vi "LowEnd-FPGA.vi"() -> ()   [LabVIEW 2016]
uses:
  Faraday Cup Readback.ctl
  Aperture Readback.ctl
  Gate Valve Readback.ctl
  Glassman Control.ctl
  Glassman Readback.ctl
  <vilib>/LabVIEW Targets/FPGA/cRIO/shared/nicrio_ModuleControls/nicrio_cRIO-9871_BaudRateEnum.ctl
  <vilib>/LabVIEW Targets/FPGA/cRIO/shared/nicrio_ModuleControls/nicrio_cRIO-9871_DataBitsEnum.ctl
  <vilib>/LabVIEW Targets/FPGA/cRIO/shared/nicrio_ModuleControls/nicrio_cRIO-9871_ParityEnum.ctl
  <vilib>/LabVIEW Targets/FPGA/cRIO/shared/nicrio_ModuleControls/nicrio_cRIO-9871_StopBitsEnum.ctl
  <vilib>/Platform/TimedLoop/XDataNode/timing_clust.ctl
  <vilib>/Platform/TimedLoop/XDataNode/nitl_modes.ctl
  <vilib>/Platform/TimedLoop/XDataNode/wakeup.ctl
  <vilib>/rvi/FXPMathLib/basic elements/FxpIntAccumulator/subVIs/nifxpmath_IntAccumulator_SimConfig.ctl
  <vilib>/rvi/Emulation/niFpgaGetClockAttributes.vi
  <vilib>/rvi/Emulation/niFpgaSctlEmulationGetInTimedLoop.vi
  <vilib>/rvi/Emulation/niFpgaEmulationReportErrorSimple.vi
  <vilib>/rvi/eio/common/nirviEmuTemplateMethod_errors.vi
  <vilib>/rvi/Emulation/niFpgaCriticalErrorInLSC.vi
  <vilib>/rvi/Analysis/common/codeGenErrors/XNode/niFpgaXNodeCodeGenErrorHandle.vi
  <vilib>/rvi/FXPMathLib/basic elements/FxpIntAccumulator/simVIs/DllFxpIntAccumulator_sub.vi
  <vilib>/rvi/eio/common/nirviEmuTemplatePropertySet_errors.vi
  <vilib>/eio/EIONode/EIONode.xnode
  <vilib>/rvi/Analysis/measure/dc-rms/XNode/niFpgaDC-RMS.xnode
  <vilib>/Platform/TimedLoop/XDataNode/XDataNode.xnode
  <vilib>/rvi/FXPMathLib/basic elements/FxpIntAccumulator/XNode/nifxpmath_IntAccumulator.xnode
  <vilib>/rvi/FXPMathLib/FxpMul/XNode/nifxpmath_Multiplier.xnode
  <vilib>/eio/EIOPropertyNode/EIOPropertyNode.xnode
  <vilib>/eio/EIOMethodNode/EIOMethodNode.xnode
  <vilib>/Platform/TimedLoop/XDataNode/XDNodeRunTimeDep.lvlib
  <vilib>/rvi/FXPMathLib/sim/FxpSim.dll
  <vilib>/rvi/eio/common/nirviEmuTemplatePropertyGet_errors.vi
  <vilib>/rvi/eio/common/nirviEmuTemplatePropertyGet_noerrors.vi
  <vilib>/rvi/eio/common/nirviEmuTemplatePropertySet_noerrors.vi
panel:
  in  "Tank Entrance Vac Interlock bypass":bool
  in  "LowEnd Waist Vac Interlock bypass":bool
  out "HV readback loop #2 error":errorcluster
  out "Tank Entrance Y2- readback":T1
  out "Tank Entrance Y2+ readback":T1
  out "Tank Entrance Y1- readback":T1
  out "Tank Entrance Y1+ readback":T1
  out "Tank Entrance X- readback":T1
  out "Tank Entrance X+ readback":T1
  out "HV readback loop #1 error":errorcluster
  out "LE Einzel readback":T1
  out "LE Waist Y- readback":T1
  out "LE Waist Y+ readback":T1
  out "LE Waist X- readback":T1
  out "LE Waist X+ readback":T1
  out "HV control loop 1 error":errorcluster
  in  "LE Einzel V set":T2
  in  "LE Waist Y- Steerer V set":T2
  in  "LE Waist Y+ Steerer V set":T2
  in  "LE Waist X- Steerer V set":T2
  in  "LE Waist X+ Steerer V set":T2
  out "HV control loop 2 error":errorcluster
  in  "Tank Entrance Y2- Steerer V set":T2
  in  "Tank Entrance Y2+ Steerer V set":T2
  in  "Tank Entrance Y1- Steerer V set":T2
  in  "Tank Entrance Y1+ Steerer V set":T2
  in  "Tank Entrance X- Steerer V set":T2
  in  "Tank Entrance X+ Steerer V set":T2
  out "LowEnd Waist Vac Interlock":bool
  out "Tank Entrance Vac Interlock":bool
  out "Turbo GV Position":T3
  out "Beamline GV Position":T3
  out "Cryo Pump GV Position":T3
  out "Bounce Mag Image \nAperture Position":T4
  out "LowEnd Waist FC Position":T5
  out "Tank Entrance FC Position":T5
  out "Actuator-sensor loop error":errorcluster
  out "GV Interlock loop error":errorcluster
  in  "Turbo GV":bool
  in  "Beamline GV":bool
  in  "Cryo Pump GV":bool
  in  "Bounce Magnet\n Image Aperture":bool
  in  "RT error":bool
  out "Tank Entrance Ion Gauge 2":u8[](array[numeric])
  out "Tank Entrance Convectron 2":u8[](array[numeric])
  out "Tank Entrance Convectron 1":u8[](array[numeric])
  out "Tank Entrance Ion Gauge 1":u8[](array[numeric])
  out "Tank Entrance Vac Gauge error":errorcluster
  out "Low End Waist Ion Gauge 2":u8[](array[numeric])
  out "Low End Waist Convectron 2":u8[](array[numeric])
  out "Low End Waist Convectron 1":u8[](array[numeric])
  out "Low End Waist Ion Gauge 1":u8[](array[numeric])
  out "Low End Waist Vac Gauge error":errorcluster
  in  "LowEnd Waist FC":bool
  in  "Tank Entrance FC":bool
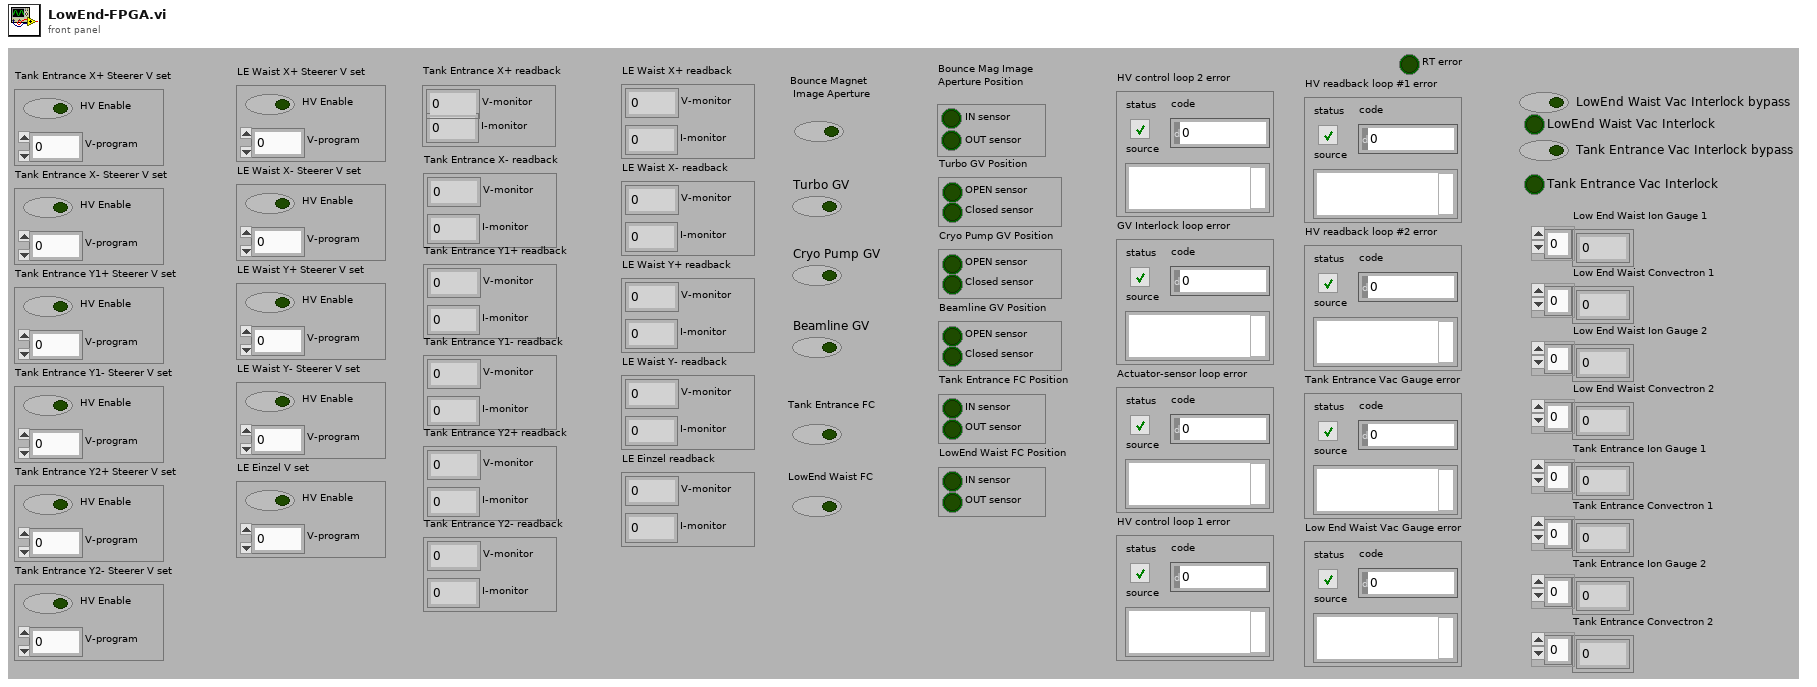
[diagram p1: front panel]
types:
  T1 = typedef "Glassman Readback.ctl" = cluster{"I-monitor":fxp<+/-,16,5>, "V-monitor":fxp<+/-,16,5>}
  T2 = typedef "Glassman Control.ctl" = cluster{"V-program":fxp<+/-,16,5>, "HV Enable":bool}
  T3 = typedef "Gate Valve Readback.ctl" = cluster{"OPEN sensor":bool, "Closed sensor":bool}
  T4 = typedef "Aperture Readback.ctl" = cluster{"IN sensor":bool, "OUT sensor":bool}
  T5 = typedef "Faraday Cup Readback.ctl" = cluster{"IN sensor":bool, "OUT sensor":bool}
  T6 = typedef "nicrio_cRIO-9871_StopBitsEnum.ctl" = enum8{"1", "1.5", "2"}
  T7 = typedef "nicrio_cRIO-9871_ParityEnum.ctl" = enum8{"None", "Odd", "Even", "Mark", "Space"}
  T8 = typedef "nicrio_cRIO-9871_DataBitsEnum.ctl" = enum8{"5", "6", "7", "8"}
  T9 = typedef "nicrio_cRIO-9871_BaudRateEnum.ctl" = enum16{"75 bps", "110 bps", "134 bps", "150 bps", "300 bps", "600 bps", "1200 bps", "1800 bps", "2400 bps", "4800 bps", "7200 bps", "9600 bps", "14.4 kbps", "19.2 kbps", "28.8 kbps", "38.4 kbps", "57.6 kbps", "115.2 kbps", "230.4 kbps", "460.8 kbps", "921.6 kbps"}
  T10 = typedef "XDNodeRunTimeDep.lvlib/timing_clust.ctl" = cluster{"Expected End [f-1]":u64, "Actual End [f-1]":u64, "Finished Late? [f-1]":bool, "Expected End [i-1]":u64, "Actual End [i-1]":u64, "Finished Late? [i-1]":bool, "Expected Start [i]":u64, "Actual Start [i]":u64, "Expected Start [f]":u64, "Actual Start [f]":u64, "Source Name":string, "Structure Name":string, "Period":i64, "Deadline":i64, "Offset":i64, "Start":i64, "Priority":i32, "Timeout":i32, "Mode":T11, "Wakeup Reason":T12, "Error":errorcluster, "Source Type":string, "Secondary Source Type":string, "Global End Time":u64, "Global Start Time":u64, "Frame Duration":u64, "Iteration Duration":u64, "Assigned CPU":i32, "I/O Scan Engine Mode":u32}
  T11 = typedef "XDNodeRunTimeDep.lvlib/nitl_modes.ctl" = enum32{"No Change", "Process missed periods, maintain original phase", "Discard missed periods, maintain original phase", "Process missed periods, ignore original phase", "Discard missed periods, ignore original phase"}
  T12 = typedef "XDNodeRunTimeDep.lvlib/wakeup.ctl" = enum32{"Normal", "Aborted", "Asynchronous wakeup", "Timing source error", "Timed loop error", "Timeout"}
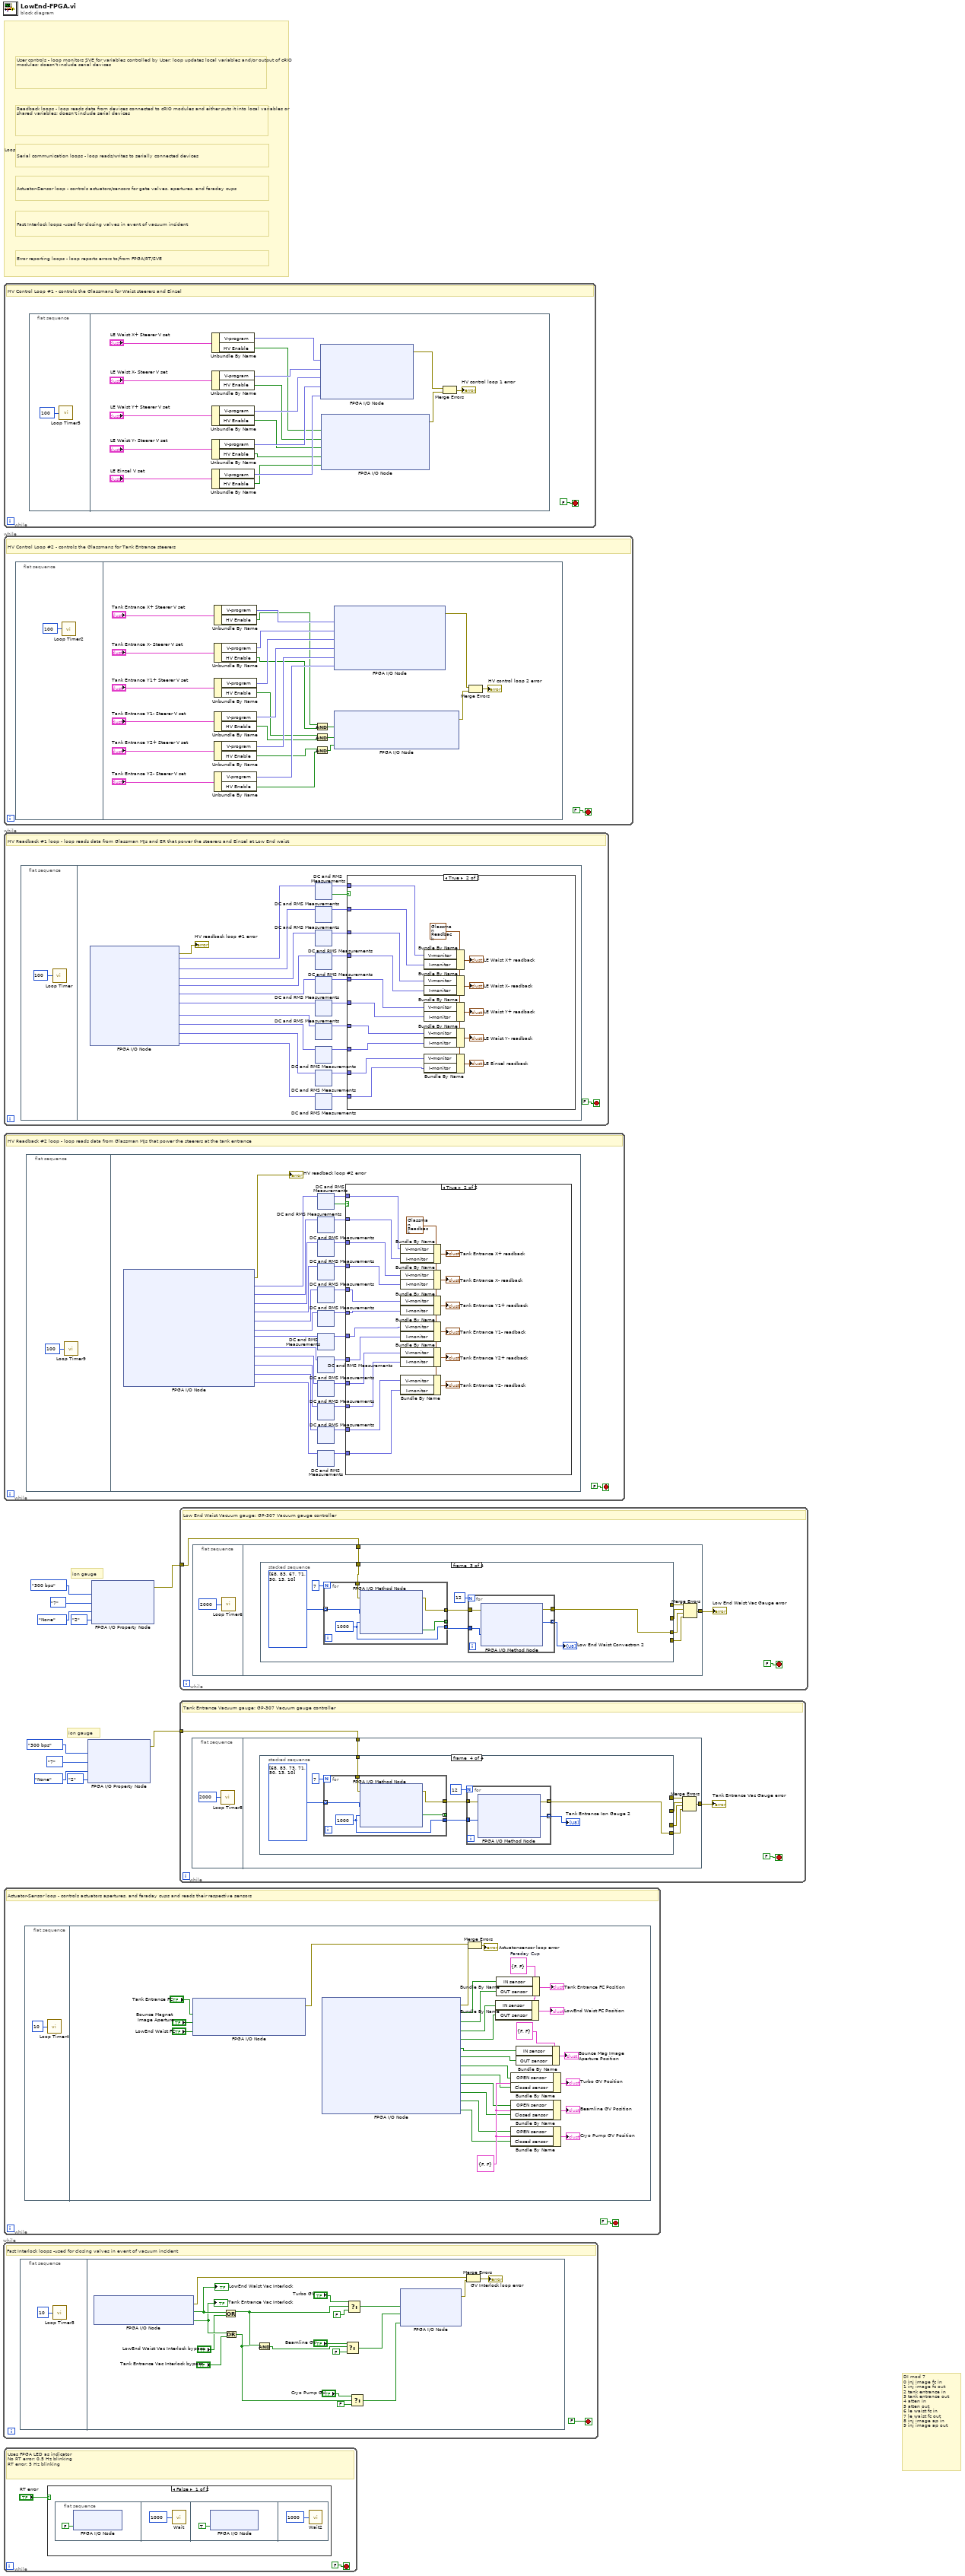
[diagram p0: block diagram]
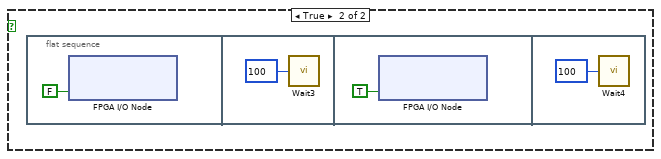
[diagram p2: hidden frame]
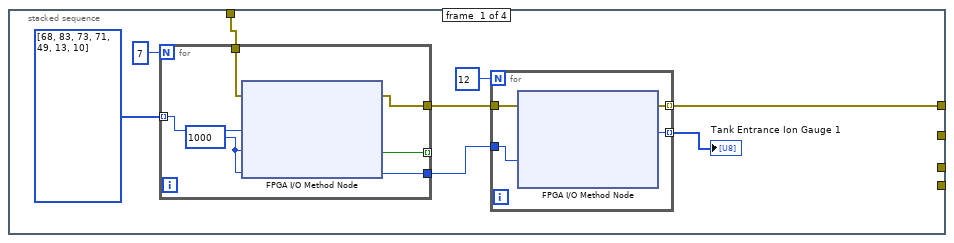
[diagram p3: hidden frame]
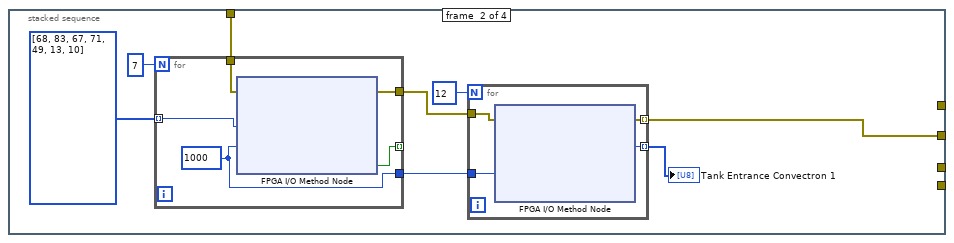
[diagram p4: hidden frame]
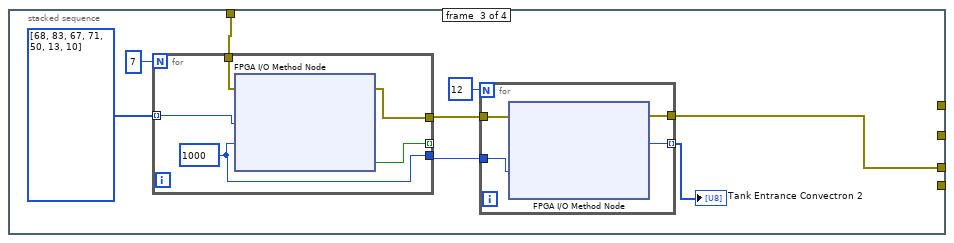
[diagram p5: hidden frame]
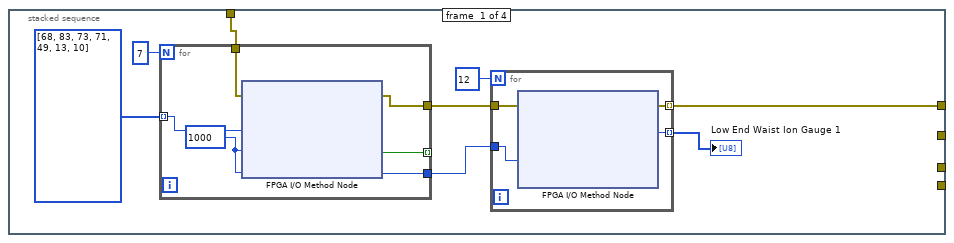
[diagram p6: hidden frame]
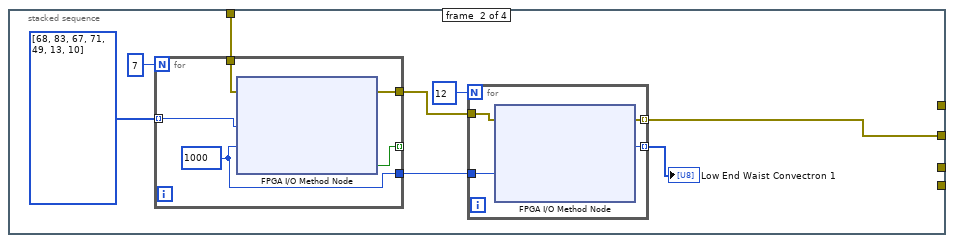
[diagram p7: hidden frame]
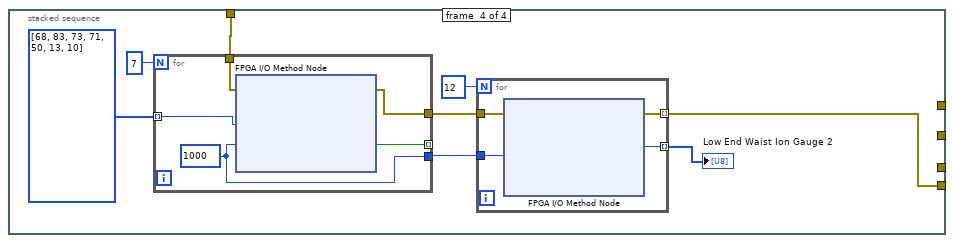
[diagram p8: hidden frame]
diagram:
  # "DI mod 7\n0 inj image fc in\n1 inj image fc out\n2 tank entrance in\n3 tank entrance out\n4 atten in\n5 atten out\n6 le waist fc in\n7 le waist fc out\n8 inj image ap in\n9 inj image ap out"
  # "Actuator-Sensor loop - controls actuators/sensors for gate valves, apertures, and faraday cups"
  # "Fast Interlock loops -used for closing valves in event of vacuum incident"
  # "Error reporting loops - loop reports errors to/from FPGA/RT/SVE"
  # "Serial communication loops - loop reads/writes to serially connected devices"
  # "Readback loops - loop reads data from devices connected to cRIO modules and either puts it into local variables or shared variables; doesn't include serial devices"
  # "User controls - loop monitors SVE for variables controlled by User; loop updates local variables and/or output of cRIO modules; doesn't include serial devices"
  # "Loop legend - loops are color coded by responsibility"
  # "ion gauge"
  # "ion gauge"
  n1 = while {
    stop <- FALSE ("stop") stop-if-true
    # "Fast Interlock loops -used for closing valves in event of vacuum incident"
    n2 = flat-sequence {
      frame #0 {
        n3 = call "Loop Timer3"("Count(uSec)"=u32 10 ("Count(Ticks)")) -> ()  [unwired: 1 out]
      }
      frame #1 {
        n4 = xnode "FPGA I/O Node"() -> ("error out"=w29:errorcluster, "LowEnd Waist Vac Interlock"=w18:bool, "Tank Entrance Vac Interlock"=w17:bool)  [unwired: 3 in, 2 out]
        "Tank Entrance Vac Interlock" <- w17
        "LowEnd Waist Vac Interlock" <- w18
        n5 = Or(x=w18, y="LowEnd Waist Vac Interlock bypass") -> (x .or. y?=w16:bool)
        n6 = Or(x=w17, y="Tank Entrance Vac Interlock bypass") -> (x .or. y?=w15:bool)
        n7 = And(x=w16, y=w15) -> (x .and. y?=w22:bool)
        n8 = Select(t="Beamline GV", s=w22, f=FALSE) -> (s? t:f=w24:bool)
        n9 = Select(t="Turbo GV", s=w16, f=FALSE) -> (s? t:f=w21:bool)
        n10 = Select(t="Cryo Pump GV", s=w15, f=FALSE) -> (s? t:f=w28:bool)
        n11 = xnode "FPGA I/O Node"("Turbo GV"=w21, "Beamline GV"=w24, "Cryo Pump GV"=w28) -> ("error out"=w30:errorcluster)  [unwired: 4 in, 3 out]
        n12 = Merge Errors(w29, w30) -> (→"GV Interlock loop error":errorcluster)
      }
    }
  }
  n13 = while {
    stop <- FALSE stop-if-true
    # "HV Control Loop #1 - controls the Glassmans for Waist steerers and Einzel"
    n14 = flat-sequence {
      frame #0 {
        n15 = call "Loop Timer5"("Count(mSec)"=u32 100) -> ()  [unwired: 1 out]
      }
      frame #1 {
        n16 = Unbundle By Name("LE Waist X+ Steerer V set") -> ("V-program"=w46:fxp<+/-,16,5>, "HV Enable"=w41:bool)
        n17 = Unbundle By Name("LE Waist X- Steerer V set") -> ("V-program"=w45:fxp<+/-,16,5>, "HV Enable"=w40:bool)
        n18 = Unbundle By Name("LE Waist Y+ Steerer V set") -> ("V-program"=w44:fxp<+/-,16,5>, "HV Enable"=w39:bool)
        n19 = Unbundle By Name("LE Waist Y- Steerer V set") -> ("V-program"=w43:fxp<+/-,16,5>, "HV Enable"=w38:bool)
        n20 = Unbundle By Name("LE Einzel V set") -> ("V-program"=w42:fxp<+/-,16,5>, "HV Enable"=w37:bool)
        n21 = xnode "FPGA I/O Node"("LE Waist X+ Steerer V set"=w46, "LE Waist X- Steerer V set"=w45, "LE Waist Y+ Steerer V set"=w44, "LE Waist Y- Steerer V set"=w43, "LE Einzel V set"=w42) -> ("error out"=w35:errorcluster)  [unwired: 6 in, 5 out]
        n22 = xnode "FPGA I/O Node"("LE Waist X+ steerer HV Enable"=w41, "LE Waist X- steerer HV Enable"=w40, "LE Waist Y+ steerer HV Enable"=w39, "LE Waist Y- steerer HV Enable"=w38, "LE Einzel HV Enable"=w37) -> ("error out"=w36:errorcluster)  [unwired: 6 in, 5 out]
        n23 = Merge Errors(w35, w36) -> (→"HV control loop 1 error":errorcluster)
      }
    }
  }
  n24 = while {
    stop <- FALSE stop-if-true
    # "HV Control Loop #2 - controls the Glassmans for Tank Entrance steerers"
    n25 = flat-sequence {
      frame #0 {
        n26 = call "Loop Timer2"("Count(mSec)"=u32 100) -> ()  [unwired: 1 out]
      }
      frame #1 {
        n27 = Unbundle By Name("Tank Entrance X+ Steerer V set") -> ("V-program"=w71:fxp<+/-,16,5>, "HV Enable"=w65:bool)
        n28 = Unbundle By Name("Tank Entrance X- Steerer V set") -> ("V-program"=w70:fxp<+/-,16,5>, "HV Enable"=w63:bool)
        n29 = Unbundle By Name("Tank Entrance Y1+ Steerer V set") -> ("V-program"=w69:fxp<+/-,16,5>, "HV Enable"=w58:bool)
        n30 = Unbundle By Name("Tank Entrance Y1- Steerer V set") -> ("V-program"=w68:fxp<+/-,16,5>, "HV Enable"=w59:bool)
        n31 = Unbundle By Name("Tank Entrance Y2+ Steerer V set") -> ("V-program"=w67:fxp<+/-,16,5>, "HV Enable"=w61:bool)
        n32 = Unbundle By Name("Tank Entrance Y2- Steerer V set") -> ("V-program"=w66:fxp<+/-,16,5>, "HV Enable"=w62:bool)
        n33 = And(x=w65, y=w63) -> (x .and. y?=w64:bool)
        n34 = And(x=w58, y=w59) -> (x .and. y?=w57:bool)
        n35 = And(x=w61, y=w62) -> (x .and. y?=w60:bool)
        n36 = xnode "FPGA I/O Node"("Tank Entrance X+ Steerer V set"=w71, "Tank Entrance X- Steerer V set"=w70, "Tank Entrance Y1+ Steerer V set"=w69, "Tank Entrance Y1- Steerer V set"=w68, "Tank Entrance Y2+ Steerer V set"=w67, "Tank Entrance Y2- Steerer V set"=w66) -> ("error out"=w55:errorcluster)  [unwired: 7 in, 6 out]
        n37 = xnode "FPGA I/O Node"("Tank Entrance X steerers HV Enable"=w64, "Tank Entrance Y1 steerers HV Enable"=w57, "Tank Entrance Y2 steerers HV Enable"=w60) -> ("error out"=w56:errorcluster)  [unwired: 4 in, 3 out]
        n38 = Merge Errors(w55, w56) -> (→"HV control loop 2 error":errorcluster)
      }
    }
  }
  n39 = while {
    stop <- FALSE stop-if-true
    # "HV Readback #1 loop - loop reads data from Glassman MJs and ER that power the steerers and Einzel at Low End waist"
    n40 = flat-sequence {
      frame #0 {
        n41 = call "Loop Timer"("Count(mSec)"=u32 100 ("Count(Ticks)")) -> ()  [unwired: 1 out]
      }
      frame #1 {
        n42 = xnode "FPGA I/O Node"() -> ("error out"=→"HV readback loop #1 error":errorcluster, "LE Waist X+ V readback"=w100:fxp<+/-,26,5>, "LE Waist X+ I readback"=w98:fxp<+/-,26,5>, "LE Waist X- V readback"=w96:fxp<+/-,26,5>, "LE Waist X- I readback"=w94:fxp<+/-,26,5>, "LE Waist Y+ V readback"=w92:fxp<+/-,26,5>, "LE Waist Y+ I readback"=w90:fxp<+/-,26,5>, "LE Waist Y- V readback"=w88:fxp<+/-,26,5>, "LE Waist Y- I readback"=w86:fxp<+/-,26,5>, "LE Einzel V readback"=w84:fxp<+/-,26,5>, "LE Einzel I readback"=w82:fxp<+/-,26,5>)  [unwired: 11 in, 10 out]
        n43 = xnode "DC and RMS Measurements"("input data"=w100) -> ("DC"=w99:fxp<+/-,26,5>, "output valid"=w101:bool)  [unwired: 1 in]
        n44 = xnode "DC and RMS Measurements"("input data"=w98) -> ("DC"=w97:fxp<+/-,26,5>)  [unwired: 1 in, 1 out]
        n45 = xnode "DC and RMS Measurements"("input data"=w96) -> ("DC"=w95:fxp<+/-,26,5>)  [unwired: 1 in, 1 out]
        n46 = xnode "DC and RMS Measurements"("input data"=w94) -> ("DC"=w93:fxp<+/-,26,5>)  [unwired: 1 in, 1 out]
        n47 = xnode "DC and RMS Measurements"("input data"=w92) -> ("DC"=w91:fxp<+/-,26,5>)  [unwired: 1 in, 1 out]
        n48 = xnode "DC and RMS Measurements"("input data"=w90) -> ("DC"=w89:fxp<+/-,26,5>)  [unwired: 1 in, 1 out]
        n49 = xnode "DC and RMS Measurements"("input data"=w88) -> ("DC"=w87:fxp<+/-,26,5>)  [unwired: 1 in, 1 out]
        n50 = xnode "DC and RMS Measurements"("input data"=w86) -> ("DC"=w85:fxp<+/-,26,5>)  [unwired: 1 in, 1 out]
        n51 = xnode "DC and RMS Measurements"("input data"=w84) -> ("DC"=w83:fxp<+/-,26,5>)  [unwired: 1 in, 1 out]
        n52 = xnode "DC and RMS Measurements"("input data"=w82) -> ("DC"=w81:fxp<+/-,26,5>)  [unwired: 1 in, 1 out]
        n53 = case shown="True" w101 {
          tunnel: w99 -> [_ w111]
          tunnel: w97 -> [_ w110]
          tunnel: w95 -> [_ w109]
          tunnel: w93 -> [_ w108]
          tunnel: w91 -> [_ w107]
          tunnel: w89 -> [_ w106]
          tunnel: w87 -> [_ w105]
          tunnel: w85 -> [_ w104]
          tunnel: w83 -> [_ w103]
          tunnel: w81 -> [_ w102]
          frame False {
          }
          frame True {
            w112 = T1 {"I-monitor"=0.0, "V-monitor"=0.0} ("Glassman Readback")
            n54 = Bundle By Name(cluster=w112, "V-monitor"=w111, "I-monitor"=w110) -> (→"LE Waist X+ readback":T1)
            n55 = Bundle By Name(cluster=w112, "V-monitor"=w109, "I-monitor"=w108) -> (→"LE Waist X- readback":T1)
            n56 = Bundle By Name(cluster=w112, "V-monitor"=w107, "I-monitor"=w106) -> (→"LE Waist Y+ readback":T1)
            n57 = Bundle By Name(cluster=w112, "V-monitor"=w105, "I-monitor"=w104) -> (→"LE Waist Y- readback":T1)
            n58 = Bundle By Name(cluster=w112, "V-monitor"=w103, "I-monitor"=w102) -> (→"LE Einzel readback":T1)
          }
        }
      }
    }
  }
  n59 = while {
    stop <- FALSE stop-if-true
    # "HV Readback #2 loop - loop reads data from Glassman MJs that power the steerers at the tank entrance"
    n60 = flat-sequence {
      frame #0 {
        n61 = call "Loop Timer9"("Count(mSec)"=u32 100 ("Count(Ticks)")) -> ()  [unwired: 1 out]
      }
      frame #1 {
        n62 = xnode "FPGA I/O Node"() -> ("error out"=→"HV readback loop #2 error":errorcluster, "Tank Entrance X+ Steerer V readback"=w944:fxp<+/-,26,5>, "Tank Entrance X+ Steerer I readback"=w942:fxp<+/-,26,5>, "Tank Entrance X- Steerer V readback"=w940:fxp<+/-,26,5>, "Tank Entrance X- Steerer I readback"=w938:fxp<+/-,26,5>, "Tank Entrance Y1+ Steerer V readback"=w936:fxp<+/-,26,5>, "Tank Entrance Y1+ Steerer I readback"=w934:fxp<+/-,26,5>, "Tank Entrance Y1- Steerer V readback"=w932:fxp<+/-,26,5>, "Tank Entrance Y1- Steerer I readback"=w930:fxp<+/-,26,5>, "Tank Entrance Y2+ Steerer V readback"=w928:fxp<+/-,26,5>, "Tank Entrance Y2+ Steerer I readback"=w926:fxp<+/-,26,5>, "Tank Entrance Y2- Steerer V readback"=w924:fxp<+/-,26,5>, "Tank Entrance Y2- Steerer I readback"=w922:fxp<+/-,26,5>)  [unwired: 13 in, 12 out]
        n63 = xnode "DC and RMS Measurements"("input data"=w944) -> ("DC"=w943:fxp<+/-,26,5>, "output valid"=w945:bool)  [unwired: 1 in]
        n64 = xnode "DC and RMS Measurements"("input data"=w942) -> ("DC"=w941:fxp<+/-,26,5>)  [unwired: 1 in, 1 out]
        n65 = xnode "DC and RMS Measurements"("input data"=w940) -> ("DC"=w939:fxp<+/-,26,5>)  [unwired: 1 in, 1 out]
        n66 = xnode "DC and RMS Measurements"("input data"=w938) -> ("DC"=w937:fxp<+/-,26,5>)  [unwired: 1 in, 1 out]
        n67 = xnode "DC and RMS Measurements"("input data"=w936) -> ("DC"=w935:fxp<+/-,26,5>)  [unwired: 1 in, 1 out]
        n68 = xnode "DC and RMS Measurements"("input data"=w934) -> ("DC"=w933:fxp<+/-,26,5>)  [unwired: 1 in, 1 out]
        n69 = xnode "DC and RMS Measurements"("input data"=w932) -> ("DC"=w931:fxp<+/-,26,5>)  [unwired: 1 in, 1 out]
        n70 = xnode "DC and RMS Measurements"("input data"=w930) -> ("DC"=w929:fxp<+/-,26,5>)  [unwired: 1 in, 1 out]
        n71 = xnode "DC and RMS Measurements"("input data"=w928) -> ("DC"=w927:fxp<+/-,26,5>)  [unwired: 1 in, 1 out]
        n72 = xnode "DC and RMS Measurements"("input data"=w926) -> ("DC"=w925:fxp<+/-,26,5>)  [unwired: 1 in, 1 out]
        n73 = xnode "DC and RMS Measurements"("input data"=w924) -> ("DC"=w923:fxp<+/-,26,5>)  [unwired: 1 in, 1 out]
        n74 = xnode "DC and RMS Measurements"("input data"=w922) -> ("DC"=w921:fxp<+/-,26,5>)  [unwired: 1 in, 1 out]
        n75 = case shown="True" w945 {
          tunnel: w943 -> [_ w957]
          tunnel: w941 -> [_ w956]
          tunnel: w939 -> [_ w955]
          tunnel: w937 -> [_ w954]
          tunnel: w935 -> [_ w953]
          tunnel: w933 -> [_ w952]
          tunnel: w931 -> [_ w951]
          tunnel: w929 -> [_ w950]
          tunnel: w927 -> [_ w949]
          tunnel: w925 -> [_ w948]
          tunnel: w923 -> [_ w947]
          tunnel: w921 -> [_ w946]
          frame False {
          }
          frame True {
            w958 = T1 {"I-monitor"=0.0, "V-monitor"=0.0} ("Glassman Readback")
            n76 = Bundle By Name(cluster=w958, "V-monitor"=w957, "I-monitor"=w956) -> (→"Tank Entrance X+ readback":T1)
            n77 = Bundle By Name(cluster=w958, "V-monitor"=w955, "I-monitor"=w954) -> (→"Tank Entrance X- readback":T1)
            n78 = Bundle By Name(cluster=w958, "V-monitor"=w953, "I-monitor"=w952) -> (→"Tank Entrance Y1+ readback":T1)
            n79 = Bundle By Name(cluster=w958, "V-monitor"=w951, "I-monitor"=w950) -> (→"Tank Entrance Y1- readback":T1)
            n80 = Bundle By Name(cluster=w958, "V-monitor"=w949, "I-monitor"=w948) -> (→"Tank Entrance Y2+ readback":T1)
            n81 = Bundle By Name(cluster=w958, "V-monitor"=w947, "I-monitor"=w946) -> (→"Tank Entrance Y2- readback":T1)
          }
        }
      }
    }
  }
  n82 = while {
    stop <- FALSE stop-if-true
    # "Actuator-Sensor loop - controls actuators apertures, and faraday cups and reads their respective sensors"
    n83 = flat-sequence {
      frame #0 {
        n84 = call "Loop Timer4"("Count(uSec)"=u32 10 ("Count(Ticks)")) -> ()  [unwired: 1 out]
      }
      frame #1 {
        w1943 = T3 {"OPEN sensor"=FALSE, "Closed sensor"=FALSE} ("Gate Valve")
        w1946 = T5 {"IN sensor"=FALSE, "OUT sensor"=FALSE}  # Faraday Cup
        n85 = xnode "FPGA I/O Node"("Tank Entrance FC"="Tank Entrance FC", "Bounce Magnet Image Aperture"="Bounce Magnet\n Image Aperture", "LowEnd Waist FC"="LowEnd Waist FC") -> ("error out"=w1928:errorcluster)  [unwired: 4 in, 3 out]
        n86 = xnode "FPGA I/O Node"() -> ("error out"=w1951:errorcluster, "Tank Entrance FC IN sensor"=w1949:bool, "Tank Entrance FC OUT sensor"=w1948:bool, "LowEnd Waist FC IN sensor"=w1945:bool, "LowEnd Waist FC OUT sensor"=w1944:bool, "Bounce Mag Image Aperture IN sensor"=w1941:bool, "Bounce Mag Image Aperture OUT sensor"=w1940:bool, "Turbo GV OPEN sensor"=w1938:bool, "Turbo GV CLOSED sensor"=w1937:bool, "Beamline GV OPEN sensor"=w1936:bool, "Beamline GV CLOSED sensor"=w1935:bool, "Cryo Pump GV OPEN sensor"=w1934:bool, "Cryo Pump GV CLOSED sensor"=w1933:bool)  [unwired: 13 in, 12 out]
        n87 = Merge Errors(w1928, w1951) -> (→"Actuator-sensor loop error":errorcluster)
        n88 = Bundle By Name(cluster=w1946, "IN sensor"=w1945, "OUT sensor"=w1944) -> (→"LowEnd Waist FC Position":T5)
        n89 = Bundle By Name(cluster=w1946, "IN sensor"=w1949, "OUT sensor"=w1948) -> (→"Tank Entrance FC Position":T5)
        n90 = Bundle By Name(cluster=w1943, "OPEN sensor"=w1938, "Closed sensor"=w1937) -> (→"Turbo GV Position":T3)
        n91 = Bundle By Name(cluster=w1943, "OPEN sensor"=w1936, "Closed sensor"=w1935) -> (→"Beamline GV Position":T3)
        n92 = Bundle By Name(cluster=w1943, "OPEN sensor"=w1934, "Closed sensor"=w1933) -> (→"Cryo Pump GV Position":T3)
        n93 = Bundle By Name(cluster=T4 {"IN sensor"=FALSE, "OUT sensor"=FALSE} ("Aperture"), "IN sensor"=w1941, "OUT sensor"=w1940) -> (→"Bounce Mag Image \nAperture Position":T4)
      }
    }
  }
  n94 = while {
    stop <- FALSE stop-if-true
    # "Uses FPGA LED as indicator\nNo RT error: 0.5 Hz blinking\nRT error: 5 Hz blinking"
    n95 = case shown="False" "RT error" {
      frame False {
        n96 = flat-sequence {
          frame #0 {
            n97 = xnode "FPGA I/O Node"("FPGA LED"=FALSE) -> ()  [unwired: 1 in, 1 out]
          }
          frame #1 {
            n98 = call "Wait"("Count(mSec)"=u16 1000) -> ()  [unwired: 1 out]
          }
          frame #2 {
            n99 = xnode "FPGA I/O Node"("FPGA LED"=TRUE) -> ()  [unwired: 1 in, 1 out]
          }
          frame #3 {
            n100 = call "Wait2"("Count(mSec)"=u16 1000) -> ()  [unwired: 1 out]
          }
        }
      }
      frame True {
        n101 = flat-sequence {
          frame #0 {
            n102 = xnode "FPGA I/O Node"("FPGA LED"=FALSE) -> ()  [unwired: 1 in, 1 out]
          }
          frame #1 {
            n103 = call "Wait3"("Count(mSec)"=u16 100) -> ()  [unwired: 1 out]
          }
          frame #2 {
            n104 = xnode "FPGA I/O Node"("FPGA LED"=TRUE) -> ()  [unwired: 1 in, 1 out]
          }
          frame #3 {
            n105 = call "Wait4"("Count(mSec)"=u16 100) -> ()  [unwired: 1 out]
          }
        }
      }
    }
  }
  n106 = xnode "FPGA I/O Property Node"("Baud Rate"=nicrio_cRIO-9871_BaudRateEnum."300 bps", "Data Bits"=nicrio_cRIO-9871_DataBitsEnum."7", "Parity"=nicrio_cRIO-9871_ParityEnum."None", "Stop Bits"=nicrio_cRIO-9871_StopBitsEnum."2") -> ("error out"=w2:errorcluster)  [unwired: 2 in, 1 out]
  n107 = xnode "FPGA I/O Property Node"("Baud Rate"=nicrio_cRIO-9871_BaudRateEnum."300 bps", "Data Bits"=nicrio_cRIO-9871_DataBitsEnum."7", "Parity"=nicrio_cRIO-9871_ParityEnum."None", "Stop Bits"=nicrio_cRIO-9871_StopBitsEnum."2") -> ("error out"=w1:errorcluster)  [unwired: 2 in, 1 out]
  n108 = while {
    tunnel: w2 -> [w1965]
    stop <- FALSE stop-if-true
    # "Tank Entrance Vacuum gauge: GP-307 Vacuum gauge controller"
    n109 = flat-sequence {
      tunnel: w1965 -> [w1973]
      tunnel: [w1968] -> w1964
      frame #0 {
        n110 = call "Loop Timer8"("Count(mSec)"=u32 2000 ("Count(Ticks)")) -> ()  [unwired: 1 out]
      }
      frame #1 {
        n111 = stacked-sequence {
          tunnel: [_ _ w2010 _] -> w1970
          tunnel: [_ _ _ w2026] -> w1969
          tunnel: w1973 -> [w1976 w1993 w2008 w2025]
          tunnel: [w1974 _ _ _] -> w1972
          tunnel: [_ w1992 _ _] -> w1971
          frame #0 {
            n112 = for {
              N: 7 -> [_]
              tunnel: [w1990] -> w1977
              tunnel: [w1989] -> _ mode=indexing
              tunnel: u8[] [68, 83, 73, 71, 49, 13, 10] ("unsigned byte array") -> [w1988] mode=indexing
              tunnel: w1976 -> [w1987]
              tunnel: [w1986] -> w1975
              w1990 = 1000 ("Timeout (ms)")
              n113 = xnode "FPGA I/O Method Node"("error in"=w1987, "Data"=w1988, "Timeout (ms)"=w1990) -> ("error out"=w1986:errorcluster, "Timed Out"=w1989:bool)  [unwired: 1 in, 1 out]
            }
            n114 = for {
              N: 12 -> [_]
              tunnel: w1977 -> [w1985]
              tunnel: [w1984] -> w1978 mode=indexing
              tunnel: w1975 -> [w1983]
              tunnel: [w1982] -> w1974 mode=indexing
              n115 = xnode "FPGA I/O Method Node"("error in"=w1983, "Timeout (ms)"=w1985) -> ("error out"=w1982:errorcluster, "Data"=w1984:u8)  [unwired: 1 in, 2 out]
            }
            "Tank Entrance Ion Gauge 1" <- w1978
          }
          frame #1 {
            n116 = for {
              N: 7 -> [_]
              tunnel: [w2006] -> w1998
              tunnel: [w2005] -> _ mode=indexing
              tunnel: u8[] [68, 83, 67, 71, 49, 13, 10] ("unsigned byte array") -> [w2007] mode=indexing
              tunnel: w1993 -> [w2004]
              tunnel: [w2003] -> w1991
              w2006 = 1000 ("Timeout (ms)")
              n117 = xnode "FPGA I/O Method Node"("error in"=w2004, "Data"=w2007, "Timeout (ms)"=w2006) -> ("error out"=w2003:errorcluster, "Timed Out"=w2005:bool)  [unwired: 1 in, 1 out]
            }
            n118 = for {
              N: 12 -> [_]
              tunnel: w1998 -> [w2002]
              tunnel: [w2001] -> w1994 mode=indexing
              tunnel: w1991 -> [w2000]
              tunnel: [w1999] -> w1992 mode=indexing
              n119 = xnode "FPGA I/O Method Node"("error in"=w2000, "Timeout (ms)"=w2002) -> ("error out"=w1999:errorcluster, "Data"=w2001:u8)  [unwired: 1 in, 2 out]
            }
            "Tank Entrance Convectron 1" <- w1994
          }
          frame #2 {
            n120 = for {
              N: 7 -> [_]
              tunnel: [w2022] -> w2015
              tunnel: [w2023] -> _ mode=indexing
              tunnel: u8[] [68, 83, 67, 71, 50, 13, 10] ("unsigned byte array") -> [w2024] mode=indexing
              tunnel: [w2021] -> w2011
              tunnel: w2008 -> [w2020]
              w2022 = 1000 ("Timeout (ms)")
              n121 = xnode "FPGA I/O Method Node"("error in"=w2020, "Data"=w2024, "Timeout (ms)"=w2022) -> ("error out"=w2021:errorcluster, "Timed Out"=w2023:bool)  [unwired: 1 in, 1 out]
            }
            n122 = for {
              N: 12 -> [_]
              tunnel: w2015 -> [w2019]
              tunnel: [w2018] -> w2009 mode=indexing
              tunnel: w2011 -> [w2017]
              tunnel: [w2016] -> w2010
              n123 = xnode "FPGA I/O Method Node"("error in"=w2017, "Timeout (ms)"=w2019) -> ("error out"=w2016:errorcluster, "Data"=w2018:u8)  [unwired: 1 in, 2 out]
            }
            "Tank Entrance Convectron 2" <- w2009
          }
          frame #3 {
            n124 = for {
              N: 7 -> [_]
              tunnel: [w2039] -> w2032
              tunnel: [w2041] -> _ mode=indexing
              tunnel: u8[] [68, 83, 73, 71, 50, 13, 10] ("unsigned byte array") -> [w2040] mode=indexing
              tunnel: [w2038] -> w2027
              tunnel: w2025 -> [w2037]
              w2039 = 1000 ("Timeout (ms)")
              n125 = xnode "FPGA I/O Method Node"("error in"=w2037, "Data"=w2040, "Timeout (ms)"=w2039) -> ("error out"=w2038:errorcluster, "Timed Out"=w2041:bool)  [unwired: 1 in, 1 out]
            }
            n126 = for {
              N: 12 -> [_]
              tunnel: w2032 -> [w2036]
              tunnel: [w2035] -> w2028 mode=indexing
              tunnel: w2027 -> [w2034]
              tunnel: [w2033] -> w2026 mode=indexing
              n127 = xnode "FPGA I/O Method Node"("error in"=w2034, "Timeout (ms)"=w2036) -> ("error out"=w2033:errorcluster, "Data"=w2035:u8)  [unwired: 1 in, 2 out]
            }
            "Tank Entrance Ion Gauge 2" <- w2028
          }
        }
        n128 = Merge Errors(w1972, w1971, w1970, w1969) -> (w1968:errorcluster)
      }
    }
    "Tank Entrance Vac Gauge error" <- w1964
  }
  n129 = while {
    tunnel: w1 -> [w2043]
    stop <- FALSE stop-if-true
    # "Low End Waist Vacuum gauge: GP-307 Vacuum gauge controller"
    n130 = flat-sequence {
      tunnel: w2043 -> [w2051]
      tunnel: [w2046] -> w2042
      frame #0 {
        n131 = call "Loop Timer6"("Count(mSec)"=u32 2000 ("Count(Ticks)")) -> ()  [unwired: 1 out]
      }
      frame #1 {
        n132 = stacked-sequence {
          tunnel: [_ _ w2088 _] -> w2048
          tunnel: [_ _ _ w2104] -> w2047
          tunnel: w2051 -> [w2054 w2071 w2086 w2103]
          tunnel: [w2052 _ _ _] -> w2050
          tunnel: [_ w2070 _ _] -> w2049
          frame #0 {
            n133 = for {
              N: 7 -> [_]
              tunnel: [w2068] -> w2055
              tunnel: [w2067] -> _ mode=indexing
              tunnel: u8[] [68, 83, 73, 71, 49, 13, 10] ("unsigned byte array") -> [w2066] mode=indexing
              tunnel: w2054 -> [w2065]
              tunnel: [w2064] -> w2053
              w2068 = 1000 ("Timeout (ms)")
              n134 = xnode "FPGA I/O Method Node"("error in"=w2065, "Data"=w2066, "Timeout (ms)"=w2068) -> ("error out"=w2064:errorcluster, "Timed Out"=w2067:bool)  [unwired: 1 in, 1 out]
            }
            n135 = for {
              N: 12 -> [_]
              tunnel: w2055 -> [w2063]
              tunnel: [w2062] -> w2056 mode=indexing
              tunnel: w2053 -> [w2061]
              tunnel: [w2060] -> w2052 mode=indexing
              n136 = xnode "FPGA I/O Method Node"("error in"=w2061, "Timeout (ms)"=w2063) -> ("error out"=w2060:errorcluster, "Data"=w2062:u8)  [unwired: 1 in, 2 out]
            }
            "Low End Waist Ion Gauge 1" <- w2056
          }
          frame #1 {
            n137 = for {
              N: 7 -> [_]
              tunnel: [w2084] -> w2076
              tunnel: [w2083] -> _ mode=indexing
              tunnel: u8[] [68, 83, 67, 71, 49, 13, 10] ("unsigned byte array") -> [w2085] mode=indexing
              tunnel: w2071 -> [w2082]
              tunnel: [w2081] -> w2069
              w2084 = 1000 ("Timeout (ms)")
              n138 = xnode "FPGA I/O Method Node"("error in"=w2082, "Data"=w2085, "Timeout (ms)"=w2084) -> ("error out"=w2081:errorcluster, "Timed Out"=w2083:bool)  [unwired: 1 in, 1 out]
            }
            n139 = for {
              N: 12 -> [_]
              tunnel: w2076 -> [w2080]
              tunnel: [w2079] -> w2072 mode=indexing
              tunnel: w2069 -> [w2078]
              tunnel: [w2077] -> w2070 mode=indexing
              n140 = xnode "FPGA I/O Method Node"("error in"=w2078, "Timeout (ms)"=w2080) -> ("error out"=w2077:errorcluster, "Data"=w2079:u8)  [unwired: 1 in, 2 out]
            }
            "Low End Waist Convectron 1" <- w2072
          }
          frame #2 {
            n141 = for {
              N: 7 -> [_]
              tunnel: [w2100] -> w2093
              tunnel: [w2101] -> _ mode=indexing
              tunnel: u8[] [68, 83, 67, 71, 50, 13, 10] ("unsigned byte array") -> [w2102] mode=indexing
              tunnel: [w2099] -> w2089
              tunnel: w2086 -> [w2098]
              w2100 = 1000 ("Timeout (ms)")
              n142 = xnode "FPGA I/O Method Node"("error in"=w2098, "Data"=w2102, "Timeout (ms)"=w2100) -> ("error out"=w2099:errorcluster, "Timed Out"=w2101:bool)  [unwired: 1 in, 1 out]
            }
            n143 = for {
              N: 12 -> [_]
              tunnel: w2093 -> [w2097]
              tunnel: [w2096] -> w2087 mode=indexing
              tunnel: w2089 -> [w2095]
              tunnel: [w2094] -> w2088
              n144 = xnode "FPGA I/O Method Node"("error in"=w2095, "Timeout (ms)"=w2097) -> ("error out"=w2094:errorcluster, "Data"=w2096:u8)  [unwired: 1 in, 2 out]
            }
            "Low End Waist Convectron 2" <- w2087
          }
          frame #3 {
            n145 = for {
              N: 7 -> [_]
              tunnel: [w2117] -> w2110
              tunnel: [w2119] -> _ mode=indexing
              tunnel: u8[] [68, 83, 73, 71, 50, 13, 10] ("unsigned byte array") -> [w2118] mode=indexing
              tunnel: [w2116] -> w2105
              tunnel: w2103 -> [w2115]
              w2117 = 1000 ("Timeout (ms)")
              n146 = xnode "FPGA I/O Method Node"("error in"=w2115, "Data"=w2118, "Timeout (ms)"=w2117) -> ("error out"=w2116:errorcluster, "Timed Out"=w2119:bool)  [unwired: 1 in, 1 out]
            }
            n147 = for {
              N: 12 -> [_]
              tunnel: w2110 -> [w2114]
              tunnel: [w2113] -> w2106 mode=indexing
              tunnel: w2105 -> [w2112]
              tunnel: [w2111] -> w2104 mode=indexing
              n148 = xnode "FPGA I/O Method Node"("error in"=w2112, "Timeout (ms)"=w2114) -> ("error out"=w2111:errorcluster, "Data"=w2113:u8)  [unwired: 1 in, 2 out]
            }
            "Low End Waist Ion Gauge 2" <- w2106
          }
        }
        n149 = Merge Errors(w2050, w2049, w2048, w2047) -> (w2046:errorcluster)
      }
    }
    "Low End Waist Vac Gauge error" <- w2042
  }
